vi "is_alfa_num.vi"(1 "char":u8) -> (0 "isAlfaNum":bool)   [LabVIEW 2011]
panel:
  out "string":string
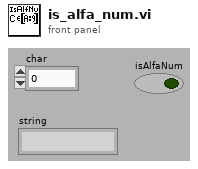
[diagram p1: front panel]
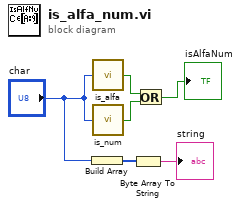
[diagram p0: block diagram]
diagram:
  n1 = Build Array("char") -> (w2:u8[])
  n2 = call "is_alfa.vi"("char"="char") -> ("isAlfa"=w5:bool)
  n3 = call "is_num.vi"("char"="char") -> ("isNum"=w4:bool)
  n4 = Byte Array To String(unsigned byte array=w2) -> (string=→"string":string)
  n5 = Or(x=w5, y=w4) -> (x .or. y?=→"isAlfaNum":bool)
